vi "ReadPowerSetting(Basic).vi"(7 "Memory":i8=1 min=1 max=50, 8 "Error In":errorcluster, 11 "VISA resource name":refnum<visa-resource-name>) -> (0 "Error Out":errorcluster, 2 "Setting":dbl, 3 "VISA resource name out":refnum<visa-resource-name>)   [LabVIEW 2013]
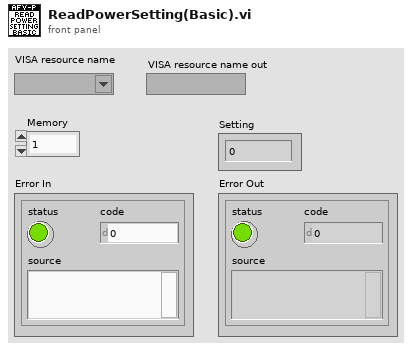
[diagram p1: front panel]
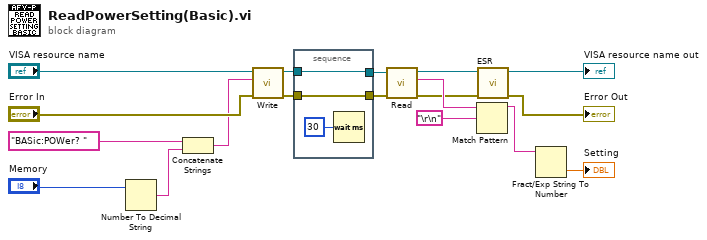
[diagram p0: block diagram]
diagram:
  n1 = Number To Decimal String(number="Memory") -> (decimal integer string=w16:string)  [unwired: 1 in]
  n2 = Concatenate Strings("BASic:POWer? " ("Write Buffer"), w16) -> (w4:string)
  n3 = call "Write.vi"("Error In"="Error In", "Write Buffer"=w4, "VISA resource name"="VISA resource name") -> ("Error Out"=w10:errorcluster, "VISA resource name out"=w13:refnum<visa-resource-name>)  [unwired: 7 in]
  n4 = stacked-sequence {
    tunnel: [w20] -> w12
    tunnel: w13 -> [w20]
    tunnel: [w19] -> w11
    tunnel: w10 -> [w19]
    frame #0 {
      n5 = Wait (ms)(milliseconds to wait=u32 30) -> ()  [unwired: 1 out]
    }
  }
  n6 = call "Read.vi"("Error In"=w11, "VISA resource name"=w12) -> ("Error Out"=w8:errorcluster, "Read Data"=w9:string, "VISA resource name out"=w7:refnum<visa-resource-name>)  [unwired: 7 in]
  n7 = Match Pattern(string=w9, regular expression="\r\n") -> (before substring=w1:string)  [unwired: 1 in, 3 out]
  n8 = call "ESR.vi"("Error In"=w8, "VISA resource name"=w7) -> ("Error Out"=→"Error Out":errorcluster, "VISA resource name out"=→"VISA resource name out":refnum<visa-resource-name>)  [unwired: 8 in]
  n9 = Fract/Exp String To Number(string=w1) -> (number=→"Setting":dbl)  [unwired: 3 in, 1 out]
